vi "Initialize.vi"(8 "error in (no error)":errorcluster, 9 "Reset (True)":bool=TRUE, 10 "ID Query (True)":bool=TRUE, 11 "VISA resource name":refnum<visa-resource-name>) -> (0 "error out":errorcluster, 3 "VISA resource name out":refnum<visa-resource-name>)   [LabVIEW 2009, in "Agilent PSG MXG Series.lvlib"]
doc: "Establishes communication with the instrument and optionally performs an instrument identification query and/or an instrument reset. It also places the instrument in a default state needed for other instrument driver operations. Therefore, call this VI before calling other instrument driver VIs for this instrument. Generally, you need to call the <B>Initialize VI</B> only once at the beginning of an application."
uses:
  Agilent PSG MXG Series.lvlib
  Private/Extended User Data.ctl
panel:
  # "(c) 2009 National Instruments.  ALL RIGHTS RESERVED."
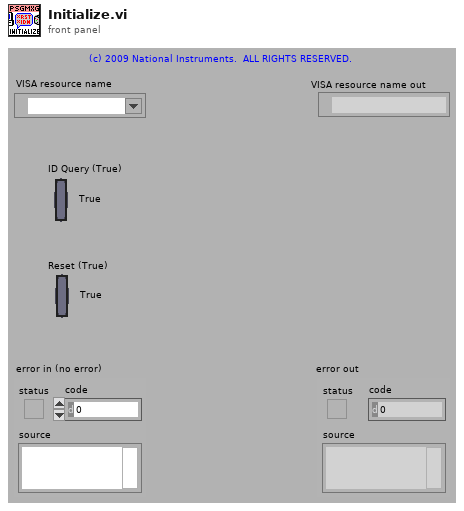
[diagram p1: front panel]
types:
  T1 = typedef "Agilent PSG MXG Series.lvlib/Extended User Data.ctl" = cluster{"Options":string[]}
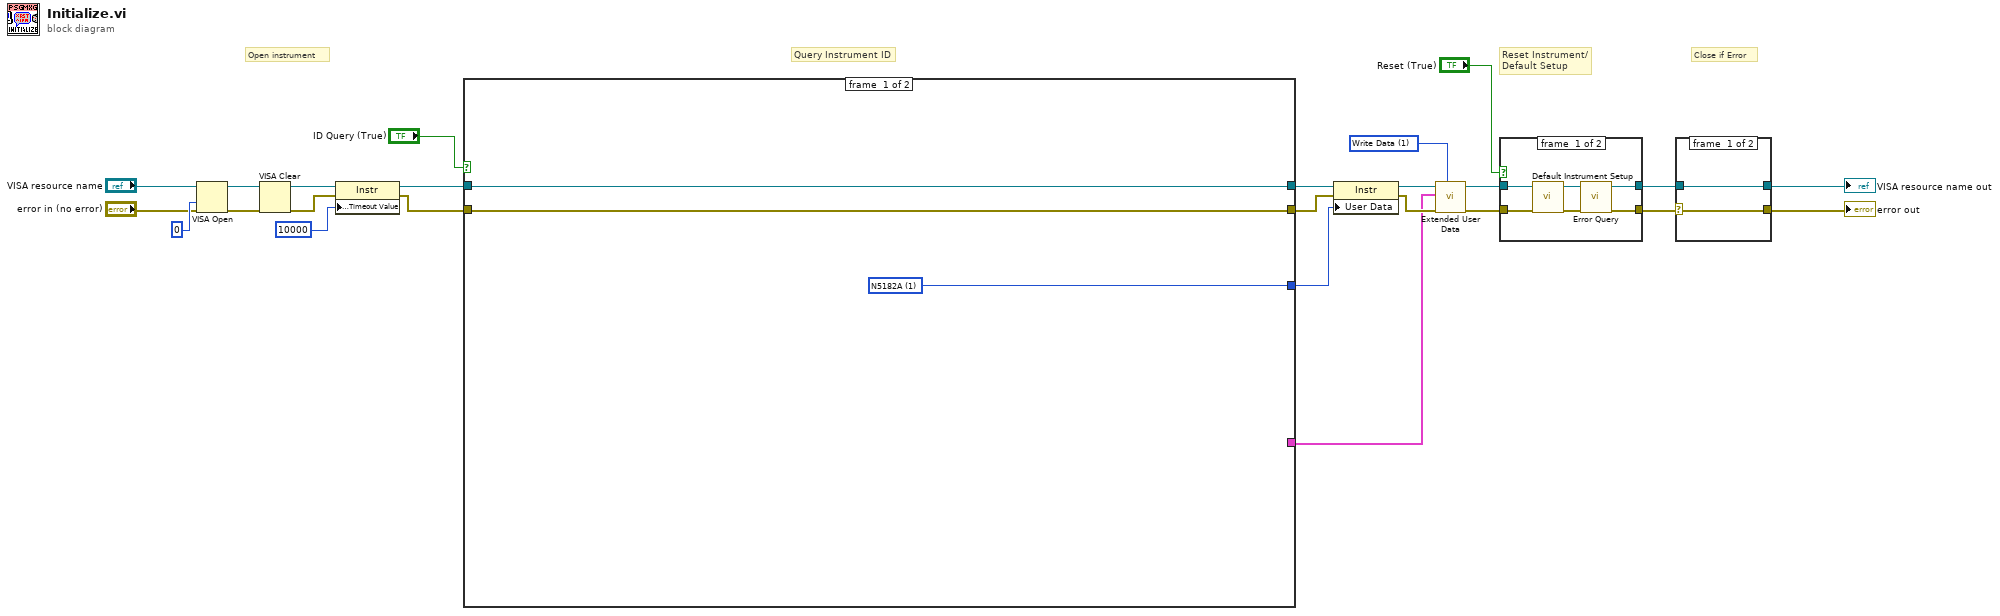
[diagram p0: block diagram]
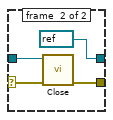
[diagram p2: hidden frame]
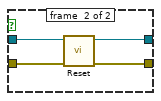
[diagram p3: hidden frame]
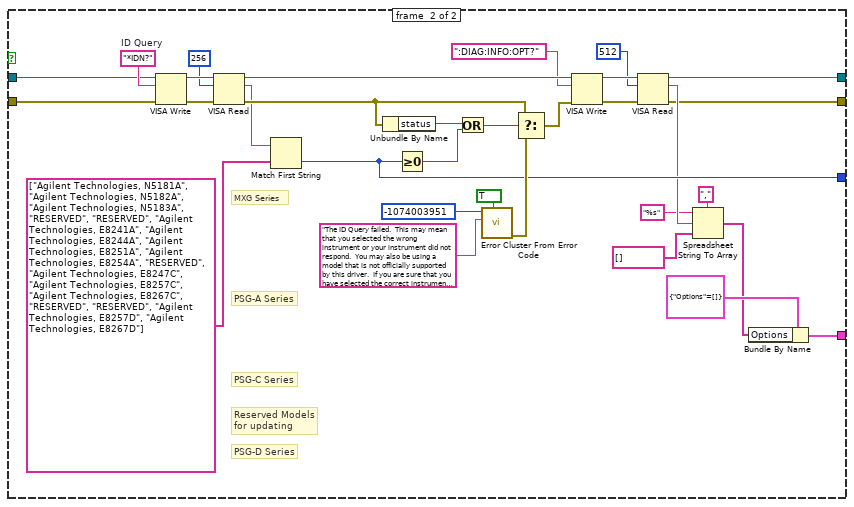
[diagram p4: hidden frame]
diagram:
  w4 = u16 1 items=["Read Data", "Write Data", "Clear Data", "Clear ALL Data"] ("Action")
  # "Close if Error"
  # "Query Instrument ID"
  # "Reset Instrument/\nDefault Setup"
  # "Open instrument"
  n1 = VISA Open(access mode=u32 0, error in (no error)="error in (no error)", VISA resource name="VISA resource name") -> (VISA resource name=w23:refnum<visa-resource-name>, error out=w22:errorcluster)  [unwired: 2 out]
  n2 = VISA Clear(VISA resource name=w23, error in (no error)=w22) -> (VISA resource name out=w21:refnum<visa-resource-name>, error out=w20:errorcluster)
  n3 = property class="Instr"(reference=w21, error in=w20, "General Settings:Timeout Value"=u32 10000) -> (reference out=w8:refnum<visa-resource-name>, error out=w7:errorcluster)
  n4 = case shown="True" "ID Query (True)" {
    tunnel: [w26 w32] -> w16
    tunnel: [w27 w33] -> w17
    tunnel: [w28 w47] -> w15
    tunnel: w8 -> [w27 w45]
    tunnel: w7 -> [w26 w44]
    tunnel: [_ w29] -> w3
    frame #0 {
      w28 = u16 1 items=["N5181A"=0, "N5182A"=1, "E8241A"=5, "E8244A"=6, "E8251A"=7, "E8254A"=8, "E8247C"=10, "E8257C"=11, "E8267C"=12, "E8257D"=15, "E8267D"=16] ("Model Type (0: N5181A)")
    }
    frame #1 {
      w57 = "*IDN?"  # ID Query
      # "Reserved Models\nfor updating"
      # "PSG-D Series"
      # "PSG-C Series"
      # "PSG-A Series"
      # "MXG Series"
      n5 = VISA Write(VISA resource name=w45, write buffer=w57, error in (no error)=w44) -> (VISA resource name out=w60:refnum<visa-resource-name>, error out=w59:errorcluster)  [unwired: 1 out]
      n6 = VISA Read(VISA resource name=w60, byte count=u32 256, error in (no error)=w59) -> (VISA resource name out=w43:refnum<visa-resource-name>, read buffer=w48:string, error out=w52:errorcluster)  [unwired: 1 out]
      n7 = Match First String(2:string[] ["Agilent Technologies, N5181A", "Agilent Technologies, N5182A", "Agilent Technologies, N5183A", "RESERVED", "RESERVED", "Agilent Technologies, E8241A", "Agilent Technologies, E8244A", "Agilent Technologies, E8251A", "Agilent Technologies, E8254A", "RESERVED", "Agilent Technologies, E8247C", "Agilent Technologies, E8257C", "Agilent Technologies, E8267C", "RESERVED", "RESERVED", "Agilent Technologies, E8257D", "Agilent Technologies, E8267D"], 3:w48) -> (0:w47:i32)  [unwired: 1 out]
      n8 = Unbundle By Name(w52) -> ("status"=w51:bool)
      n9 = Greater Or Equal To 0?(x=w47) -> (x >= 0?=w49:bool)
      n10 = Or(x=w51, y=w49) -> (x .or. y?=w50:bool)
      n11 = call <vilib>:"Error Cluster From Error Code.vi"("show call chain? (False)"=TRUE, "error message (\"\")"="The ID Query failed.  This may mean that you selected the wrong instrument or your instrument did not respond.  You may also be using a model that is not officially supported by this driver.  If you are sure that you have selected the correct instrument and it is responding, try disabling the ID Query." ("Source (VI Name)"), "error code (0)"=-1074003951 ("Code")) -> ("error out"=w56:errorcluster)  [unwired: 1 in, 5 out]
      n12 = Select(t=w52, s=w50, f=w56) -> (s? t:f=w42:errorcluster)
      n13 = VISA Write(VISA resource name=w43, write buffer=":DIAG:INFO:OPT?", error in (no error)=w42) -> (VISA resource name out=w40:refnum<visa-resource-name>, error out=w39:errorcluster)  [unwired: 1 out]
      n14 = VISA Read(VISA resource name=w40, byte count=u32 512, error in (no error)=w39) -> (VISA resource name out=w33:refnum<visa-resource-name>, read buffer=w37:string, error out=w32:errorcluster)  [unwired: 1 out]
      n15 = Spreadsheet String To Array(delimiter (Tab)=",", format string="%s", spreadsheet string=w37, array type (2D Dbl)=string[] []) -> (array=w30:string[])
      n16 = Bundle By Name(cluster=T1 {"Options"=[]} ("User Data Out"), "Options"=w30) -> (w29:T1)
    }
  }
  n17 = property class="Instr"(reference=w17, error in=w16, "User Data"=w15) -> (reference out=w6:refnum<visa-resource-name>, error out=w5:errorcluster)
  n18 = call "Extended User Data.vi"("Action"=w4, "error in (no error)"=w5, "User Data In"=w3, "VISA resource name"=w6) -> ("error out"=w1:errorcluster, "VISA resource name out"=w2:refnum<visa-resource-name>)  [unwired: 6 out]
  n19 = case shown="True" "Reset (True)" {
    tunnel: w1 -> [w65 w67]
    tunnel: [w61 w70] -> w18
    tunnel: w2 -> [w66 w68]
    tunnel: [w62 w69] -> w19
    frame #0 {
      n20 = call "Default Instrument Setup.vi"("error in (no error)"=w65, "VISA resource name"=w66) -> ("error out"=w63:errorcluster, "VISA resource name out"=w64:refnum<visa-resource-name>)  [unwired: 8 out]
      n21 = call "Error Query.vi"("error in (no error)"=w63, "VISA resource name"=w64) -> ("error out"=w61:errorcluster, "VISA resource name out"=w62:refnum<visa-resource-name>)  [unwired: 8 out]
    }
    frame #1 {
      n22 = call "Reset.vi"("error in (no error)"=w67, "VISA resource name"=w68) -> ("error out"=w70:errorcluster, "VISA resource name out"=w69:refnum<visa-resource-name>)  [unwired: 8 out]
    }
  }
  n23 = case shown="No Error" w18 {
    selector: w18 -> [w71 w74]
    tunnel: w19 -> [w72 w75]
    tunnel: [w72 refnum<visa-resource-name> refnum ("VISA resource name out")] -> w10
    tunnel: [w71 w76] -> w9
    frame #0 {
    }
    frame #1 {
      n24 = call "Close.vi"("error in (no error)"=w74, "VISA resource name"=w75) -> ("error out"=w76:errorcluster)  [unwired: 9 out]
    }
  }
  "VISA resource name out" <- w10
  "error out" <- w9
